vi "ATS9350_SimpleAsyncDMA_TR.vi"() -> ()   [LabVIEW 2010]
uses:
  ATS_ctl/ATS_DMA_Channel.ctl
  ATS_ctl/Device_Ctrl.ctl
  ATS_ctl/ATS_Check_Ctrl.ctl
  ATS_ctl/ClockSource.ctl
  ATS_ctl/ClockEdge.ctl
  ATS_ctl/Coupling.ctl
  ATS_ctl/TriggerOperation.ctl
  ATS_ctl/Bandwidth.ctl
  ATS_ctl/ExtTrigRange.ctl
  ATS_ctl/Impedance.ctl
  ATS_ctl/ATS_Async_Ctrl.ctl
  ATS_ctl/ATS_Async_Setting.ctl
  ATS_ctl/ATS_Async_Mode.ctl
  ATS_ctl/ATS_ReadSamples.ctl
panel:
  in  "Channel select":T1
  in  "stop":bool
  in  "9350 ClckRate":u32(ring)=16 items=["1 kS/s", "2 kS/s", "5 kS/s", "10 kS/s", "20 kS/s", "50 kS/s", "100 kS/s", "200 kS/s", "500 kS/s", "1 MS/s", "2 MS/s", "5 MS/s", "10 MS/s", "20 MS/s", "50 MS/s", "100 MS/s", "250 MS/s", "500 MS/s"]
  in  "Start Capture":bool
  out "Valid":bool
  out "Get Data Status":string
  out "StartCapture Status":string
  out "SetupDMA Status":string
  out "cFlags_Out":u32 format="%x"
  in  "Device Settings":bool
  in  "Samples/record":u32=1152
  in  "Records/buffer":u32=10
  out "Board":string="ATS9350"
  in  "Device":i32
  out "Waveform Graph":u16[](graph)
  # "ATS9350 Simple AsynchronousDMA VI that illustrates traditional AutoDMA acquisition"
  # "Manual"
  # "Preset"
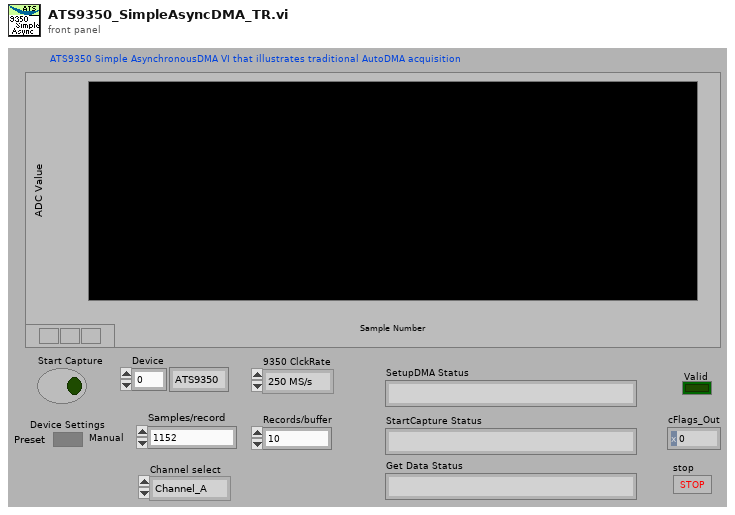
[diagram p1: front panel]
types:
  T1 = typedef "ATS_DMA_Channel.ctl" = enum16{"Channel_A", "Channel_B", "A & B"}
  T2 = typedef "ATS_Async_Ctrl.ctl" = enum16{"SetupDMA", "StartCapture", "Get", "Get_Stream", "Abort", "Stop"}
  T3 = typedef "Impedance.ctl" = enum16{"1M ohms", "50 ohms"}
  T4 = cluster{"Source":enum32{"Chan_A", "Chan_B", "External", "Disable"}, "Slope":enum32{"Positive", "Negative"}, "Level":u32}
  T5 = typedef "Coupling.ctl" = enum16{"AC", "DC"}
  T6 = typedef "ExtTrigRange.ctl" = enum16{"1 V", "5 V", "TTL"}
  T7 = typedef "Bandwidth.ctl" = enum16{"Full Bandwidth", "Reduce Bandwidth"}
  T8 = typedef "TriggerOperation.ctl" = enum16{"Only X", "Only Y", "X or Y", "X and Y", "X xor Y", "X and not Y", "not X and Y"}
  T9 = typedef "ClockEdge.ctl" = u16
  T10 = typedef "ClockSource.ctl" = enum16{"Internal", "External", "Medium Ext.", "Slow Ext.", "Ext. AC", "Ext. DC", "Ext. (PLL)"}
  T11 = typedef "ATS_Check_Ctrl.ctl" = enum16{"None", "NO_ATS9462", "ATS9462_Traditional", "Verify Board", "OnBoard Memory", "Board & Memory", "Master/Slave", "NO Master/Slave"}
  T12 = typedef "Device_Ctrl.ctl" = enum16{"Status", "About", "Arm", "ForceTrig", "Abort", "Initialize", "Init (NoPreset)", "Info", "Close", "Calibrate", "SetManually", "LED_ON", "LED_OFF"}
  T13 = cluster{"ClckSource":T10, "9350 ClckRate":u32, "ClckEdge":T9, "Decimation":u32}
  T14 = cluster{"Coupling":T5, "9350 Range":u32, "9350 Impedance":T3, "Bandwidth":T7}
  T15 = typedef "Device_Info.ctl" = cluster{"Handle":u32, "Board":string, "CPLD":string, "MemorySize":u32, "SampleSize":u8, "ID":i32, "High_Memory":bool, "Chan/Board":u8}
  T16 = cluster{"Engine Relationship":T8, "Timeout (s)":dbl, "Trig. Delay":u32, "EngineX":cluster{"Source":enum32{"Chan_A", "Chan_B", "External", "Disable"}, "Slope":enum32{"Positive", "Negative"}, "Level":u32}, "EngineY":cluster{"Source":enum32{"Chan_A", "Chan_B", "External", "Disable"}, "Slope":enum32{"Positive", "Negative"}, "Level":u32}, "Ext Trig":cluster{"Coupling":T5, "Range":T6}}
  T17 = cluster{"Count":cluster{"Count":u32, "Offset":i32, "Length":u32}, cluster{"ClckSource":T10, "9350 ClckRate":u32, "ClckEdge":T9, "Decimation":u32}, cluster{"Coupling":T5, "9350 Range":u32, "9350 Impedance":T3, "Bandwidth":T7}, cluster{"Coupling":T5, "9350 Range":u32, "9350 Impedance":T3, "Bandwidth":T7}, cluster{"Engine Relationship":T8, "Timeout (s)":dbl, "Trig. Delay":u32, "EngineX":cluster{"Source":enum32{"Chan_A", "Chan_B", "External", "Disable"}, "Slope":enum32{"Positive", "Negative"}, "Level":u32}, "EngineY":cluster{"Source":enum32{"Chan_A", "Chan_B", "External", "Disable"}, "Slope":enum32{"Positive", "Negative"}, "Level":u32}, "Ext Trig":cluster{"Coupling":T5, "Range":T6}}}
  T18 = typedef "ATS_Global.ctl" = cluster{"Record":T19, "Clock":T20, "Input A":T22, "Input B":T22, "Trigger":T24}
  T19 = typedef "Record.ctl" = cluster{"Count":u32, "Presize":u32, "Length":u32}
  T20 = typedef "Clock.ctl" = cluster{"ClckSource":T10, "ClckRate":T21, "ClckEdge":T9, "Decimation":u32}
  T21 = typedef "ClockRate.ctl" = u32
  T22 = typedef "InputCtrl.ctl" = cluster{"Coupling":T5, "Range":T23, "Impedance":T3, "Bandwidth":T7}
  T23 = typedef "Range.ctl" = u32
  T24 = typedef "Trigger.ctl" = cluster{"TrigOperation":T8, "Timeout (s)":dbl, "Trig. Delay":u32, "Engine X":T25, "Engine Y":T25, "ExtTrigControl":T26}
  T25 = typedef "TriggerEngine.ctl" = cluster{"Source":enum32{"Chan_A", "Chan_B", "External", "Disable"}, "Slope":enum32{"Positive", "Negative"}, "Level":u32}
  T26 = typedef "ExtTrigger.ctl" = cluster{"Coupling":T5, "Range":T6}
  T27 = typedef "ATS_Async_Setting.ctl" = cluster{"UseHeader":u32, "Rec/Buffer":u32, "Total_Rec":u32, "DataBuffer":bool, "GetProcessedData":bool}
  T28 = typedef "ATS_Async_Mode.ctl" = enum16{"Continuous", "Triggered", "No-Pre-Trigger", "Traditional"}
  T29 = typedef "ATS_ReadSamples.ctl" = cluster{"Offset":i32, "Length":u32}
  T30 = typedef "ATS_Async_Status.ctl" = cluster{"Start DMA":bool, "StartCapture":bool, "Valid":bool, "Completed":bool, "InProgress":bool, "Timeout":bool, "Overflow":bool, "Error":bool}
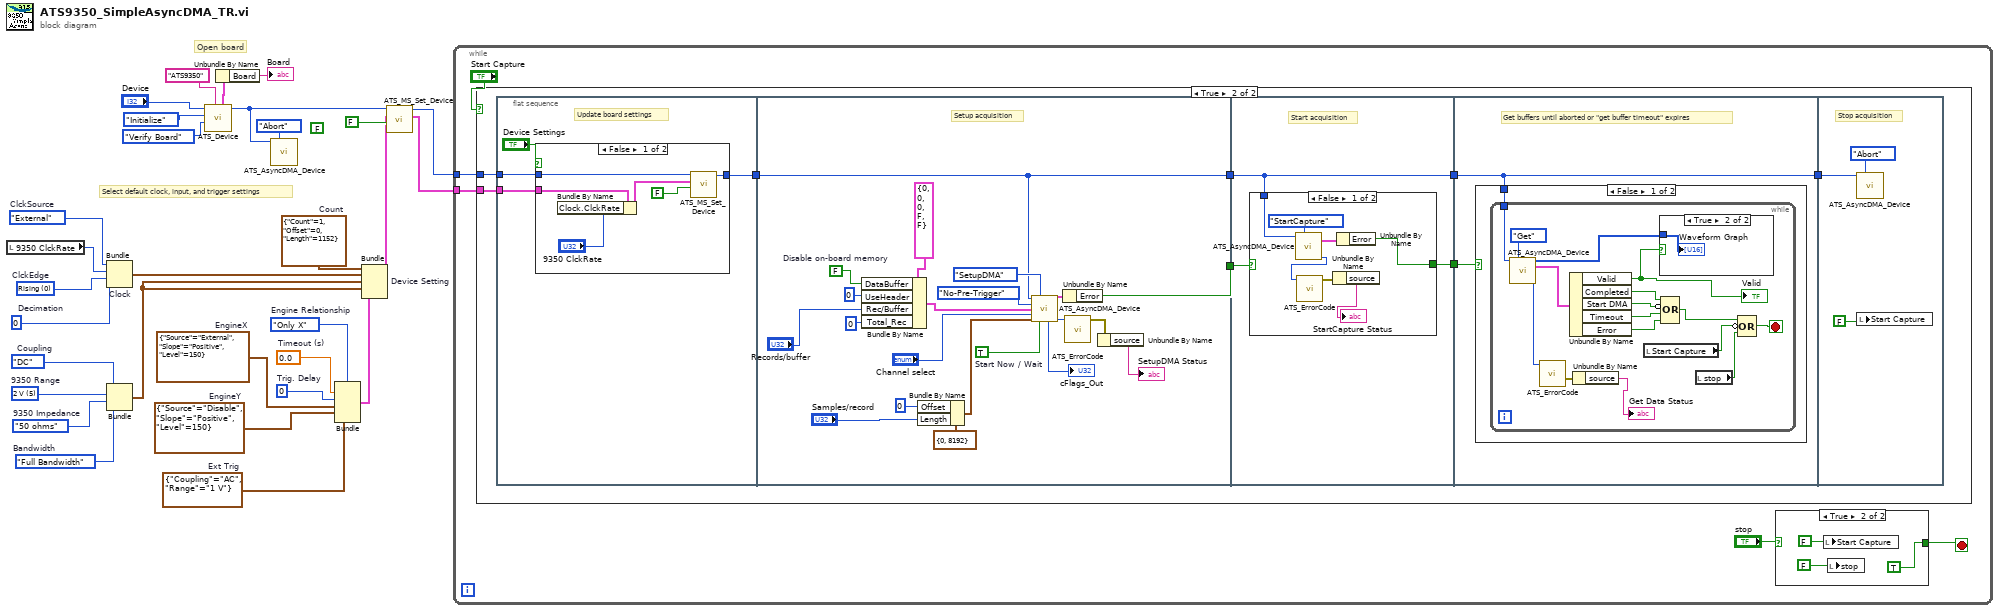
[diagram p0: block diagram]
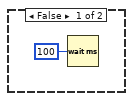
[diagram p3: hidden frame]
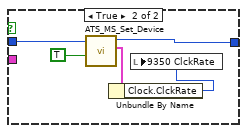
[diagram p4: hidden frame]
diagram:
  w1 = u32 5 items=["40mV", "100mV", "200mV", "400mV", "1 V", "2 V", "4 V"]  # 9350 Range
  (unwired) FALSE ("Set_Manually (F)")
  w5 = Impedance."50 ohms"  # 9350 Impedance
  w10 = T4 {"Source"=enum."Disable", "Slope"=enum."Positive", "Level"=150}  # EngineY
  w11 = T4 {"Source"=enum."External", "Slope"=enum."Positive", "Level"=150}  # EngineX
  w12 = cluster{"Coupling":T5, "Range":T6} {"Coupling"=enum."AC", "Range"=enum."1 V"}  # Ext Trig
  w13 = cluster{"Count":u32, "Offset":i32, "Length":u32} {"Count"=1, "Offset"=0, "Length"=1152}  # Count
  w14 = Bandwidth."Full Bandwidth"  # Bandwidth
  w15 = u32 0  # Decimation
  w23 = u32 0  # Trig. Delay
  w22 = TriggerOperation."Only X"  # Engine Relationship
  w24 = 0.0  # Timeout (s)
  w19 = Coupling."DC"  # Coupling
  w20 = T9 0 items=["Rising", "Falling"]  # ClckEdge
  w21 = ClockSource."External"  # ClckSource
  # "Open board"
  # "Select default clock, input, and trigger settings"
  n1 = local read "9350 ClckRate"() -> (w4:u32)
  n2 = Bundle "Clock"("ClckSource"=w21, "9350 ClckRate"=w4, "ClckEdge"=w20, "Decimation"=w15) -> (w17:T13)  [unwired: 1 in]
  n3 = Bundle("Coupling"=w19, "9350 Range"=w1, "9350 Impedance"=w5, "Bandwidth"=w14) -> (w18:T14)  [unwired: 1 in]
  n4 = call "ATS_Device.vi"("BoardToVerify"="ATS9350", "ATS_Check"=ATS_Check_Ctrl."Verify Board", "DevCtrl"=Device_Ctrl."Initialize", "DeviceIn"="Device") -> ("DeviceOut"=w2:i32, "DevInfo"=w25:T15)  [unwired: 1 in, 5 out]
  n5 = Unbundle By Name(w25) -> ("Board"=→"Board":string)
  n6 = call "ATS_AsyncDMA_Device.vi"("DeviceIn"=w2, "ATS_Async_Ctrl"=ATS_Async_Ctrl."Abort" ("ATS_DMA_Ctrl")) -> ()  [unwired: 9 in, 5 out]
  n7 = Bundle("Engine Relationship"=w22, "Timeout (s)"=w24, "Trig. Delay"=w23, "EngineX"=w11, "EngineY"=w10, "Ext Trig"=w12) -> (w16:T16)  [unwired: 1 in]
  n8 = Bundle "Device Setting"("Count"=w13, w17, w18, w18, w16) -> (w8:T17)  [unwired: 1 in]
  n9 = call "ATS_MS_Set_Device.vi"("Set_Manually (F)"=FALSE, "Setup_In"=w8, "DeviceIn"=w2) -> ("Setup_Out"=w6:T18, "DeviceOut"=w7:i32)  [unwired: 3 in, 4 out]
  n10 = while {
    tunnel: w7 -> [w35]
    tunnel: w6 -> [w33]
    stop <- w31 stop-if-true
    n11 = case shown="True" "Start Capture" {
      tunnel: w35 -> [_ w48]
      tunnel: w33 -> [_ w47]
      frame False {
        n12 = Wait (ms)(milliseconds to wait=u32 100) -> ()  [unwired: 1 out]
      }
      frame True {
        n13 = flat-sequence {
          tunnel: w47 -> [w51]
          tunnel: w48 -> [w49]
          tunnel: [w50] -> w46
          tunnel: w46 -> [w66]
          tunnel: [w66] -> w45
          tunnel: [w65] -> w43
          tunnel: w45 -> [w86]
          tunnel: [w86] -> w44
          tunnel: w43 -> [w87]
          tunnel: [w85] -> w42
          tunnel: w44 -> [w96]
          tunnel: w42 -> [w97]
          tunnel: [w96] -> w41
          tunnel: w41 -> [w117]
          frame #0 {
            # "Update board settings"
            n14 = case shown="False" "Device Settings" {
              tunnel: w49 -> [w53 w59]
              tunnel: [w57 w62] -> w50
              tunnel: w51 -> [w56 _]
              frame False {
                n15 = Bundle By Name(cluster=w56, "Clock.ClckRate"="9350 ClckRate") -> (w55:T18)
                n16 = call "ATS_MS_Set_Device.vi"("Set_Manually (F)"=FALSE, "Setup_In"=w55, "DeviceIn"=w53) -> ("DeviceOut"=w57:i32)  [unwired: 3 in, 5 out]
              }
              frame True {
                n17 = call "ATS_MS_Set_Device.vi"("Set_Manually (F)"=TRUE, "DeviceIn"=w59) -> ("Setup_Out"=w61:T18, "DeviceOut"=w62:i32)  [unwired: 4 in, 4 out]
                n18 = Unbundle By Name(w61) -> ("Clock.ClckRate"=w60:T21)
                n19 = local write "9350 ClckRate"(w60) -> ()
              }
            }
          }
          frame #1 {
            w84 = FALSE  # Disable on-board memory
            w70 = TRUE  # Start Now / Wait
            # "Setup acquisition"
            n20 = Bundle By Name(cluster=T27 {"UseHeader"=0, "Rec/Buffer"=0, "Total_Rec"=0, "DataBuffer"=FALSE, "GetProcessedData"=FALSE} ("Async_Setting"), "DataBuffer"=w84, "UseHeader"=u32 0, "Rec/Buffer"="Records/buffer", "Total_Rec"=u32 0 ("Records")) -> (w71:T27)
            n21 = Bundle By Name(cluster=T29 {"Offset"=0, "Length"=8192} ("Trad_ReadSamples"), "Offset"=0, "Length"="Samples/record") -> (w75:T29)
            n22 = call "ATS_AsyncDMA_Device.vi"("DeviceIn"=w66, "ATS_Async_Ctrl"=ATS_Async_Ctrl."SetupDMA" ("ATS_DMA_Ctrl"), "Async_Mode"=ATS_Async_Mode."No-Pre-Trigger", "Async_Setting"=w71, "Channel"="Channel select", "ReadSamples"=w75, "Start Now / Wait"=w70) -> ("Async_Status"=w79:T30, "cFlags_Out"=→"cFlags_Out":u32, "Return Code"=w81:u32)  [unwired: 4 in, 2 out]
            n23 = Unbundle By Name(w79) -> ("Error"=w65:bool)
            n24 = call "ATS_ErrorCode.vi"("ErrorCode"=w81) -> ("error out"=w80:errorcluster)  [unwired: 6 in]
            n25 = Unbundle By Name(w80) -> ("source"=→"SetupDMA Status":string)
          }
          frame #2 {
            # "Start acquisition"
            n26 = case shown="False" w87 {
              selector: w87 -> [_ w95]
              tunnel: w86 -> [w89 _]
              tunnel: [w88 w95] -> w85
              frame False {
                n27 = call "ATS_AsyncDMA_Device.vi"("DeviceIn"=w89, "ATS_Async_Ctrl"=ATS_Async_Ctrl."StartCapture") -> ("Async_Status"=w91:T30, "Return Code"=w93:u32)  [unwired: 9 in, 3 out]
                n28 = call "ATS_ErrorCode.vi"("ErrorCode"=w93) -> ("error out"=w92:errorcluster)  [unwired: 6 in]
                n29 = Unbundle By Name(w92) -> ("source"=→"StartCapture Status":string)
                n30 = Unbundle By Name(w91) -> ("Error"=w88:bool)
              }
              frame True {
              }
            }
          }
          frame #3 {
            # "Get buffers until aborted or \"get buffer timeout\" expires"
            n31 = case shown="False" w97 {
              tunnel: w96 -> [w98 _]
              frame False {
                n32 = while {
                  tunnel: w98 -> [w106]
                  stop <- w99 stop-if-true
                  n33 = call "ATS_AsyncDMA_Device.vi"("DeviceIn"=w106, "ATS_Async_Ctrl"=ATS_Async_Ctrl."Get") -> ("Buffer"=w107:u16[], "Async_Status"=w110:T30, "Return Code"=w103:u32)  [unwired: 9 in, 2 out]
                  n34 = call "ATS_ErrorCode.vi"("ErrorCode"=w103) -> ("error out"=w105:errorcluster)  [unwired: 6 in]
                  n35 = Unbundle By Name(w110) -> ("Valid"=w108:bool, "Completed"=w112:bool, "Start DMA"=w114:bool, "Timeout"=w113:bool, "Error"=w111:bool)
                  "Valid" <- w108
                  n36 = Unbundle By Name(w105) -> ("source"=→"Get Data Status":string)
                  n37 = local read "Start Capture"() -> (w101:bool)
                  n38 = case shown="True" w108 {
                    tunnel: w107 -> [_ w115]
                    frame False {
                    }
                    frame True {
                      "Waveform Graph" <- w115
                    }
                  }
                  n39 = Compound Arithmetic op=OR(w112, invert w114, w113, w111) -> (w102:bool)
                  n40 = local read "stop"() -> (w100:bool)
                  n41 = Compound Arithmetic op=OR(w102, invert w101, w100) -> (w99:bool)
                }
              }
              frame True {
              }
            }
          }
          frame #4 {
            # "Stop acquisition"
            n42 = call "ATS_AsyncDMA_Device.vi"("DeviceIn"=w117, "ATS_Async_Ctrl"=ATS_Async_Ctrl."Abort" ("ATS_DMA_Ctrl")) -> ()  [unwired: 9 in, 5 out]
            n43 = local write "Start Capture"(FALSE ("Start Capture")) -> ()
          }
        }
      }
    }
    n44 = case shown="True" "stop" {
      selector: "stop" -> [w36 _]
      tunnel: [w36 TRUE] -> w31
      frame False {
      }
      frame True {
        n45 = local write "Start Capture"(FALSE ("Start Capture")) -> ()
        n46 = local write "stop"(FALSE ("Start Capture")) -> ()
      }
    }
  }
